vi "EPTx.vi"(8 "error in (no error)":errorcluster, 11 "Node Ptr":T5 format="%.0x") -> (0 "error out":errorcluster)   [LabVIEW 2016, in "DCM System Explorer.lvlib"]
uses:
  DCM System Explorer.lvlib
  <vilib>/NI Veristand/Custom Device API/Custom Device Item Ref.ctl
  Shared/Types/EPTx RevA RT Configuration.ctl
  <vilib>/Powertrain Controls/Device Drivers/Engine Position Tracking/EPTx/RevA/RT/Controls/EPTxFilters.ctl
  Shared/Types/EPTx Signal Select.ctl
  <vilib>/Powertrain Controls/Device Drivers/DCM/Rev0/FPGA/Digital Channel.ctl
  Shared/DCM Properties.vi
  Shared/DCM Constants and GUIDs.vi
  <vilib>/NI Veristand/Custom Device Tools/Custom Device Utility Library/NI VeriStand - Search for Item by Name.vi
  <vilib>/NI VeriStand/Custom Device API/Custom Device API.lvlib
  DCM Shared.lvlib
  <vilib>/NI Veristand/Custom Device Tools/Custom Device Utility Library/Custom Device Utility Library.lvlib
  <vilib>/Powertrain Controls/Device Drivers/DCM/Rev0/FPGA/DCM - FPGA.lvlib
  <vilib>/Powertrain Controls/Device Drivers/Engine Position Tracking/EPTx/RevA/RT/EPTx - RevA - RT.lvlib
panel:
  in  "Sim Speed":sgl caption="[RPM]"
  in  "Sim Enable":bool
  in  "_Open EPTx DB Editor":bool
  in  "EPTx Signal Select":T1={"Primary"=enum."Diff IO 1", "Aux 1"=enum."Diff IO 1", "Aux 2"=enum."Diff IO 1", "Aux 3"=enum."Diff IO 1", "Aux 4"=enum."Diff IO 1"}
  in  "EPTx Configuration":T3={"EPTx Configuration Filename"="4Str_60m2_Lvl.EPTx", "StallSpeed"=200.0, "HistoryCAD"=63, "EPTxFilters"={"Primary [s]"=0.0, "Aux 1 [s]"=0.0, "Aux 2 [s]"=0.0, "Aux 3 [s]"=0.0, "Aux 4 [s]"=0.0}} {"EPTxFilters"."Aux 4 [s]" format="%#_6p"; "EPTxFilters"."Aux 3 [s]" format="%#_6p"; "EPTxFilters"."Aux 2 [s]" format="%#_6p"; "EPTxFilters"."Aux 1 [s]" format="%#_6p"; "EPTxFilters"."Primary [s]" format="%#_6p"}
  in  "Sync Enable":bool
  in  "Header":cluster{"Section Name":string}={"Section Name"="EPTx Initial Settings"}
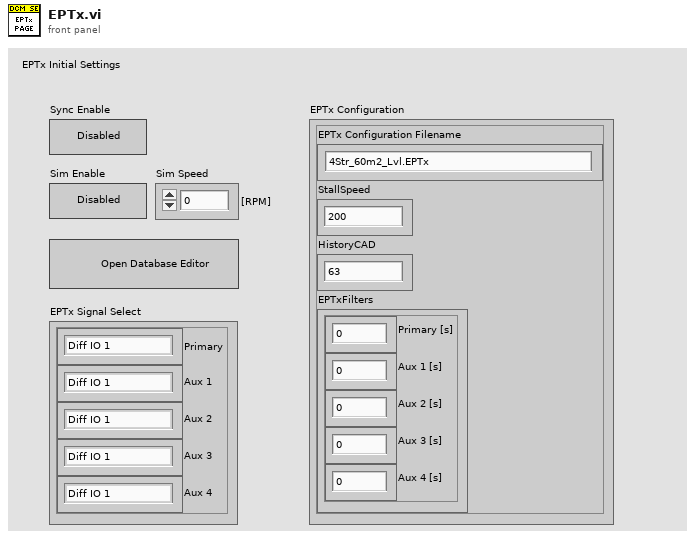
[diagram p1: front panel]
types:
  T1 = typedef "DCM Shared.lvlib/EPTx Signal Select.ctl" = cluster{"Primary":T2, "Aux 1":T2, "Aux 2":T2, "Aux 3":T2, "Aux 4":T2}
  T2 = typedef "DCM - FPGA.lvlib/Digital Channel.ctl" = enum8{"Unused", "User OS", "Diff IO 1", "Diff IO 2", "Diff IO 3", "Diff IO 4", "Diff IO 5", "Diff IO 6", "Diff IO 7", "Diff IO 8", "Aux 1", "Aux 2", "Aux 3", "Aux 4", "Aux 5", "Aux 6", "Aux 7", "Aux 8", "Aux 9", "Aux 10", "Aux 11", "Aux 12", "Aux 13", "Aux 14", "Aux 15", "Aux 16"}
  T3 = typedef "DCM Shared.lvlib/EPTx RevA RT Configuration.ctl" = cluster{"EPTx Configuration Filename":string, "StallSpeed":dbl, "HistoryCAD":u8, "EPTxFilters":T4}
  T4 = typedef "EPTx - RevA - RT.lvlib/EPTxFilters.ctl" = cluster{"Primary [s]":sgl, "Aux 1 [s]":sgl, "Aux 2 [s]":sgl, "Aux 3 [s]":sgl, "Aux 4 [s]":sgl}
  T5 = typedef "Custom Device API.lvlib/Custom Device Item Ref.ctl" = u64
  T6 = typedef "DCM Shared.lvlib/Channel.ctl" = cluster{"Name":string, "Units":string, "Default":dbl, "Description":string}
  T7 = typedef "Custom Device API.lvlib/Custom Device Channel.ctl" = cluster{"Type":T8, "Units":string, "Default Value":dbl, "Faultable":bool, "Scalable":bool}
  T8 = typedef "Custom Device API.lvlib/Custom Device Channel Type.ctl" = enum16{"Input", "Output"}
  T9 = typedef "Custom Device API.lvlib/Custom Device Commands.ctl" = enum16{"Default", "Item renamed", "Shutdown", "Dynamic button pressed"}
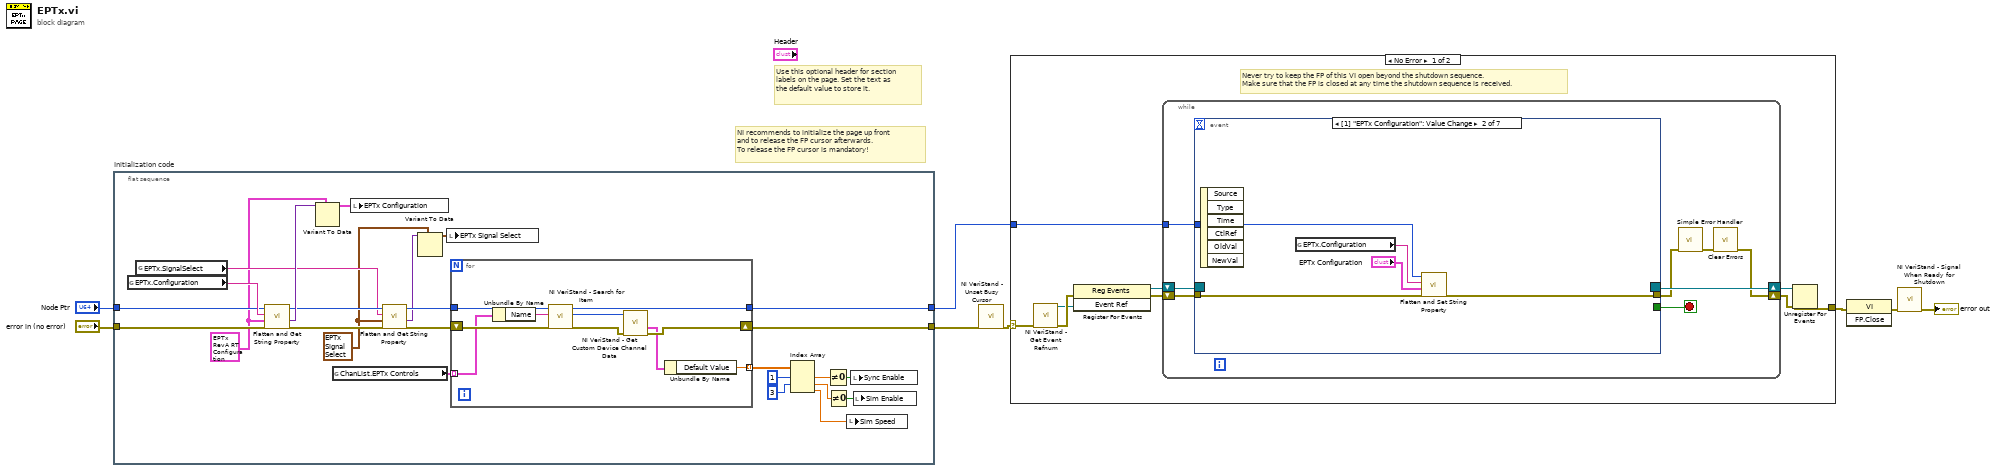
[diagram p0: block diagram]
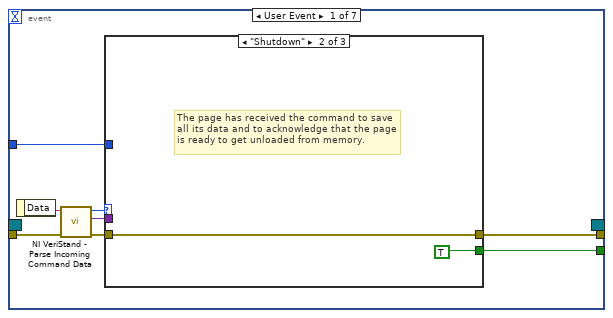
[diagram p2: hidden frame]
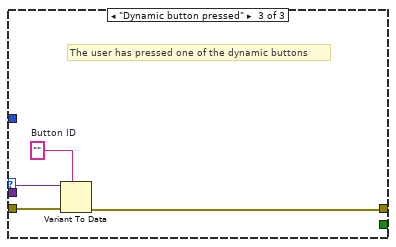
[diagram p4: hidden frame]
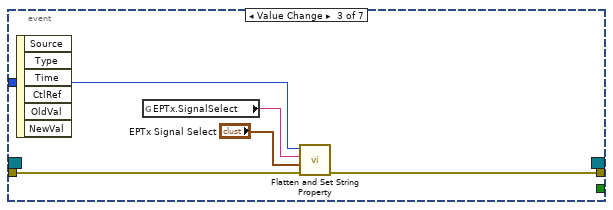
[diagram p5: hidden frame]
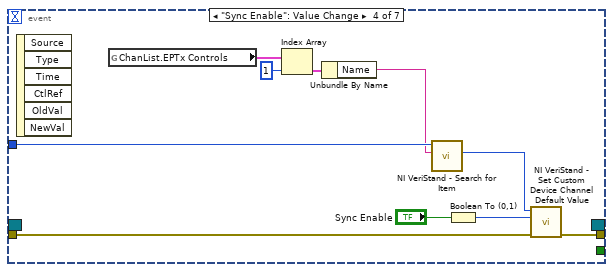
[diagram p6: hidden frame]
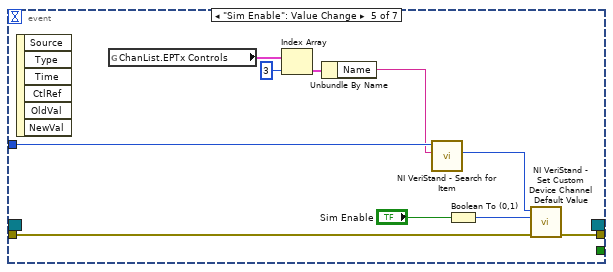
[diagram p7: hidden frame]
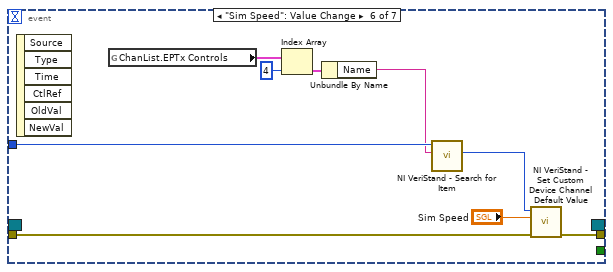
[diagram p8: hidden frame]
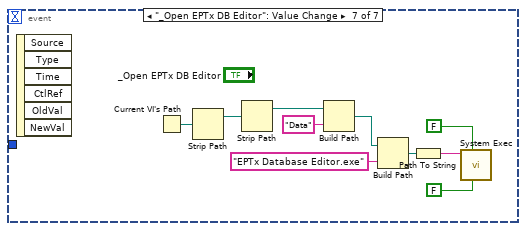
[diagram p9: hidden frame]
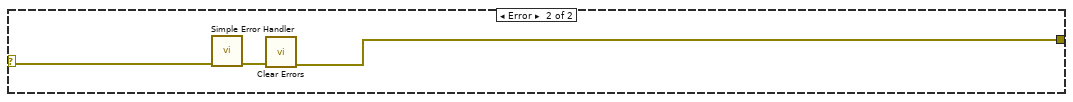
[diagram p10: hidden frame]
diagram:
  # "Use this optional header for section labels on the page. Set the text as the default value to store it."
  # "NI recommends to initialize the page up front\nand to release the FP cursor afterwards.\nTo release the FP cursor is mandatory!"
  n1 = flat-sequence "Initialization code" {
    tunnel: [w33] -> w1
    tunnel: [w32] -> w4
    tunnel: "Node Ptr" -> [w30]
    tunnel: "error in (no error)" -> [w29]
    frame #0 {
      w13 = T3 {"EPTx Configuration Filename"="4Str_60m2_Lvl.EPTx", "StallSpeed"=200.0, "HistoryCAD"=63, "EPTxFilters"={"Primary [s]"=0.0, "Aux 1 [s]"=0.0, "Aux 2 [s]"=0.0, "Aux 3 [s]"=0.0, "Aux 4 [s]"=0.0}} ("EPTx Configuration")
      w15 = T1 {"Primary"=enum."Diff IO 1", "Aux 1"=enum."Diff IO 1", "Aux 2"=enum."Diff IO 1", "Aux 3"=enum."Diff IO 1", "Aux 4"=enum."Diff IO 1"} ("EPTx Signal Select")
      n2 = global read "DCM Properties.vi" "EPTx.Configuration"() -> (w31:string)
      n3 = global read "DCM Properties.vi" "EPTx.SignalSelect"() -> (w17:string)
      n4 = call "Flatten and Get String Property.vi"("error in (no error)"=w29, "Default Value"=w13, "Property Name"=w31, "Section Ref in"=w30) -> ("error out"=w21:errorcluster, "Value"=w28:variant, "Section Ref out"=w19:T5)  [unwired: 5 in]
      n5 = Variant To Data(type=w13, Variant=w28) -> (data=w27:T3)  [unwired: 1 in, 1 out]
      n6 = global read "DCM Constants and GUIDs.vi" "ChanList.EPTx Controls"() -> (w22:T6[])
      n7 = local write "EPTx Configuration"(w27) -> ()
      n8 = call "Flatten and Get String Property.vi"("error in (no error)"=w21, "Default Value"=w15, "Property Name"=w17, "Section Ref in"=w19) -> ("error out"=w20:errorcluster, "Value"=w16:variant, "Section Ref out"=w18:T5)  [unwired: 5 in]
      n9 = Variant To Data(type=w15, Variant=w16) -> (data=w14:T1)  [unwired: 1 in, 1 out]
      n10 = local write "EPTx Signal Select"(w14) -> ()
      n11 = for {
        tunnel: w18 -> [w43]
        tunnel: [w41] -> w33
        shift-right: [w36] -> w32
        shift-left: w20 -> [w42]
        tunnel: w22 -> [w40] mode=indexing
        tunnel: [w34] -> w26 mode=indexing
        n12 = Unbundle By Name(w40) -> ("Name"=w39:string)
        n13 = call-poly <vilib>:"NI VeriStand - Search for Item.vi"("error in"=w42, "Item Name"=w39, "Section Ref in"=w43) -> ("error out"=w38:errorcluster, "Item Ref"=w37:T5, "Section Ref out"=w41:T5)  [unwired: 5 in, 1 out]
        n14 = call <vilib>:"NI VeriStand - Get Custom Device Channel Data.vi"("error in (no error)"=w38, "Channel Ref in"=w37) -> ("error out"=w36:errorcluster, "Channel"=w35:T7)  [unwired: 4 in, 4 out]
        n15 = Unbundle By Name(w35) -> ("Default Value"=w34:dbl)
      }
      n16 = Index Array(array=w26, index #1=1 ("index"), index #2=3 ("index")) -> (element #1=w24:dbl, element #2=w11:dbl, element #3=w9:dbl)  [unwired: 1 in]
      n17 = Not Equal To 0?(x=w24) -> (x != 0?=w23:bool)
      n18 = Not Equal To 0?(x=w11) -> (x != 0?=w12:bool)
      n19 = local write "Sim Speed"(w9) -> ()
      n20 = local write "Sync Enable"(w23) -> ()
      n21 = local write "Sim Enable"(w12) -> ()
    }
  }
  n22 = call <vilib>:"NI VeriStand - Unset Busy Cursor.vi"("error in (no error)"=w4) -> ("error out"=w3:errorcluster)  [unwired: 10 out]
  n23 = case shown="No Error" w3 {
    selector: w3 -> [w44 w127]
    tunnel: [w49 w125] -> w8
    tunnel: w1 -> [w45 _]
    frame No Error {
      # "Never try to keep the FP of this VI open beyond the shutdown sequence.\nMake sure that the FP is closed at any time the shutdown sequence is received."
      n24 = call <vilib>:"NI VeriStand - Get Event Refnum.vi"("error in (no error)"=w44) -> ("error out"=w52:errorcluster, "Event Ref"=w48:refnum<user-event>)  [unwired: 9 out]
      n25 = register-events(error in=w52, w48) -> (reference out=w46:refnum<event-registration>, error out=w47:errorcluster)  [unwired: 1 in]
      n26 = while {
        tunnel: w45 -> [w56]
        shift-right: [w53] -> w50
        shift-left: w47 -> [w59]
        shift-right: [w60] -> w51
        shift-left: w46 -> [w58]
        stop <- w57 stop-if-true
        n27 = event shown="[1] \"EPTx Configuration\": Value Change" {
          selector: w58 -> [_ _ _ _ _ _ _]
          dyn-events: [_ _ _ _ _ _ _] -> w60
          timeout: _ -> [_ _ _ _ _ _ _]
          tunnel: w59 -> [w68 w79 w84 w95 w105 w114 _]
          tunnel: [w64 _ _ _ _ _ _] -> w57
          tunnel: [w63 w78 w83 w94 w104 w113 _] -> w55
          tunnel: w56 -> [w62 w80 w85 w93 w103 w112 _]
          event User Event {
            n28 = event-data() -> ("Data"=w67:string)  [unwired: 1 out]
            n29 = call <vilib>:"NI VeriStand - Parse Incoming Command Data.vi"("error in (no error)"=w68, "Incoming data"=w67) -> ("error out"=w66:errorcluster, "Outgoing data"=w61:variant, "Action"=w65:T9)  [unwired: 7 out]
            n30 = case shown="\"Shutdown\"" w65 {
              tunnel: w66 -> [w69 w70 w75]
              tunnel: [_ TRUE _] -> w64
              tunnel: [w69 w70 w72] -> w63
              tunnel: w62 -> [_ _ _]
              tunnel: w61 -> [_ _ w74]
              frame "Default", Default {
              }
              frame "Shutdown" {
                # "The page has received the command to save all its data and to acknowledge that the page is ready to get unloaded from memory."
              }
              frame "Dynamic button pressed" {
                w73 = ""  # Button ID
                # "The user has pressed one of the dynamic buttons"
                n31 = Variant To Data(error in=w75, type=w73, Variant=w74) -> (error out=w72:errorcluster)  [unwired: 1 out]
              }
            }
          }
          event Value Change {
            n32 = event-data() -> ()  [unwired: 7 out]
            n33 = global read "DCM Properties.vi" "EPTx.Configuration"() -> (w76:string)
            n34 = call "Flatten and Set String Property.vi"("error in (no error)"=w79, "Value"="EPTx Configuration", "Property Name"=w76, "Section Ref in"=w80) -> ("error out"=w78:errorcluster)  [unwired: 6 in, 1 out]
          }
          event Value Change {
            n35 = event-data() -> ()  [unwired: 7 out]
            n36 = global read "DCM Properties.vi" "EPTx.SignalSelect"() -> (w82:string)
            n37 = call "Flatten and Set String Property.vi"("error in (no error)"=w84, "Value"="EPTx Signal Select", "Property Name"=w82, "Section Ref in"=w85) -> ("error out"=w83:errorcluster)  [unwired: 6 in, 1 out]
          }
          event "Sync Enable": Value Change {
            n38 = event-data() -> ()  [unwired: 7 out]
            n39 = global read "DCM Constants and GUIDs.vi" "ChanList.EPTx Controls"() -> (w91:T6[])
            n40 = Index Array(array=w91, index=1) -> (element=w89:T6)
            n41 = Unbundle By Name(w89) -> ("Name"=w88:string)
            n42 = call-poly <vilib>:"NI VeriStand - Search for Item.vi"("Item Name"=w88, "Section Ref in"=w93) -> ("Item Ref"=w92:T5)  [unwired: 6 in, 3 out]
            n43 = Boolean To (0,1)(Boolean="Sync Enable") -> (0, 1=w86:i16)
            n44 = call <vilib>:"NI VeriStand - Set Custom Device Channel Default Value.vi"("error in (no error)"=w95, "Default Value"=w86, "Channel Ref in"=w92) -> ("error out"=w94:errorcluster)  [unwired: 7 in, 1 out]
          }
          event "Sim Enable": Value Change {
            n45 = event-data() -> ()  [unwired: 7 out]
            n46 = global read "DCM Constants and GUIDs.vi" "ChanList.EPTx Controls"() -> (w101:T6[])
            n47 = Index Array(array=w101, index=3) -> (element=w99:T6)
            n48 = Unbundle By Name(w99) -> ("Name"=w98:string)
            n49 = call-poly <vilib>:"NI VeriStand - Search for Item.vi"("Item Name"=w98, "Section Ref in"=w103) -> ("Item Ref"=w102:T5)  [unwired: 6 in, 3 out]
            n50 = Boolean To (0,1)(Boolean="Sim Enable") -> (0, 1=w97:i16)
            n51 = call <vilib>:"NI VeriStand - Set Custom Device Channel Default Value.vi"("error in (no error)"=w105, "Default Value"=w97, "Channel Ref in"=w102) -> ("error out"=w104:errorcluster)  [unwired: 7 in, 1 out]
          }
          event "Sim Speed": Value Change {
            n52 = event-data() -> ()  [unwired: 7 out]
            n53 = global read "DCM Constants and GUIDs.vi" "ChanList.EPTx Controls"() -> (w110:T6[])
            n54 = Index Array(array=w110, index=4) -> (element=w108:T6)
            n55 = Unbundle By Name(w108) -> ("Name"=w107:string)
            n56 = call-poly <vilib>:"NI VeriStand - Search for Item.vi"("Item Name"=w107, "Section Ref in"=w112) -> ("Item Ref"=w111:T5)  [unwired: 6 in, 3 out]
            n57 = call <vilib>:"NI VeriStand - Set Custom Device Channel Default Value.vi"("error in (no error)"=w114, "Default Value"="Sim Speed", "Channel Ref in"=w111) -> ("error out"=w113:errorcluster)  [unwired: 7 in, 1 out]
          }
          event "_Open EPTx DB Editor": Value Change {
            n58 = event-data() -> ()  [unwired: 7 out]
            n59 = Current VI's Path() -> (path=w124:path)
            n60 = Strip Path(path=w124) -> (stripped path=w118:path)  [unwired: 1 out]
            n61 = Strip Path(path=w118) -> (stripped path=w117:path)  [unwired: 1 out]
            n62 = Build Path(base path=w117, name or relative path="Data") -> (appended path=w115:path)
            n63 = Build Path(base path=w115, name or relative path="EPTx Database Editor.exe") -> (appended path=w119:path)
            n64 = Path To String(path=w119) -> (string=w122:string)
            n65 = call <vilib>:"System Exec.vi"("run minimized? (F)"=FALSE, "wait until completion? (T)"=FALSE, "command line"=w122) -> ()  [unwired: 5 in, 4 out]
          }
        }
        n66 = call <vilib>:"Simple Error Handler.vi"("error in (no error)"=w55) -> ("error out"=w54:errorcluster)  [unwired: 1 in, 7 out]
        n67 = call <vilib>:"Clear Errors.vi"("error in (no error)"=w54) -> ("error out"=w53:errorcluster)  [unwired: 1 in, 5 out]
      }
      n68 = Unregister For Events(event registration refnum=w51, error in=w50) -> (error out=w49:errorcluster)
    }
    frame Error {
      n69 = call <vilib>:"Simple Error Handler.vi"("error in (no error)"=w127) -> ("error out"=w126:errorcluster)  [unwired: 1 in, 7 out]
      n70 = call <vilib>:"Clear Errors.vi"("error in (no error)"=w126) -> ("error out"=w125:errorcluster)  [unwired: 1 in, 5 out]
    }
  }
  n71 = invoke class="VI" method="FP.Close"(error in=w8) -> (error out=w7:errorcluster)  [unwired: 2 in, 2 out]
  n72 = call <vilib>:"NI VeriStand - Signal When Ready for Shutdown.vi"("error in (no error)"=w7) -> ("error out"=→"error out":errorcluster)  [unwired: 10 out]
